vi "AeroTestBench.vi"() -> ()   [LabVIEW 2015]
uses:
  <vilib>/Utility/file.llb/Write To Spreadsheet File (DBL).vi
panel:
  in  "amp offset":dbl
  out "error out":errorcluster
  out "Attached":bool
  out "pulses in":i32
  out "ms":dbl
  out "Total Count:":i64
  out "Total Time (ms):":dbl
  out "Frequency (Hz):":dbl format="%#_6p"
  in  "Enabled":bool
  in  "Filter:":i32(ring)=1 items=["Zero Crossing"=1, "Logic Level"=2]
  in  "Timeout (ms):":i32=100
  in  "RPM:":i32 min=0 max=1 step=1
  in  "DataRate 2":i32(slide)=128 min=8 max=1000 step=8 scale=8.0..1000.0
  in  "stop":bool
  in  "Power":bool
  out "Amperage":dbl(knob) scale=0.0..80.0
  out "Voltage":dbl(knob) scale=0.0..30.0
  out "Enable":bool
  in  "Prop Blades":u8=2
  out "RPM":dbl(knob) scale=0.0..3000.0
  out "Power Electrical":dbl(knob) scale=0.0..1000.0
  out "Boolean 2":bool
  out "Effiency":dbl(knob) scale=0.0..100.0
  out "Power Mech":dbl(knob) scale=0.0..1000.0
  out "?":bool
  in  "Save data?":bool
  in  "Path":path
  in  "File Name":string
  out "Torque":dbl(knob) scale=-5.0..5.0
  out "Thrust":dbl(knob) scale=0.0..10.0
  in  "Gain":i32(ring)=6 items=["1"=1, "8"=2, "16"=3, "32"=4, "64"=5, "128"=6]
  in  "DataRate":i32(slide)=128 min=8 max=1000 step=8 scale=8.0..1000.0
  in  "Channel 3":i32(ring)=2 items=["0", "1", "2", "3"]
  in  "Channel 2":i32(ring)=1 items=["0", "1", "2", "3"]
  in  "Channel":i32(ring) items=["0", "1", "2", "3"]
  in  "Enable":bool
  out "Actives":i32
  out "Serial":i32
  out "Active":bool
  # "Arduino"
  # "(End with .csv)"
  # "(Should be 3+)"
  # "Phidgets"
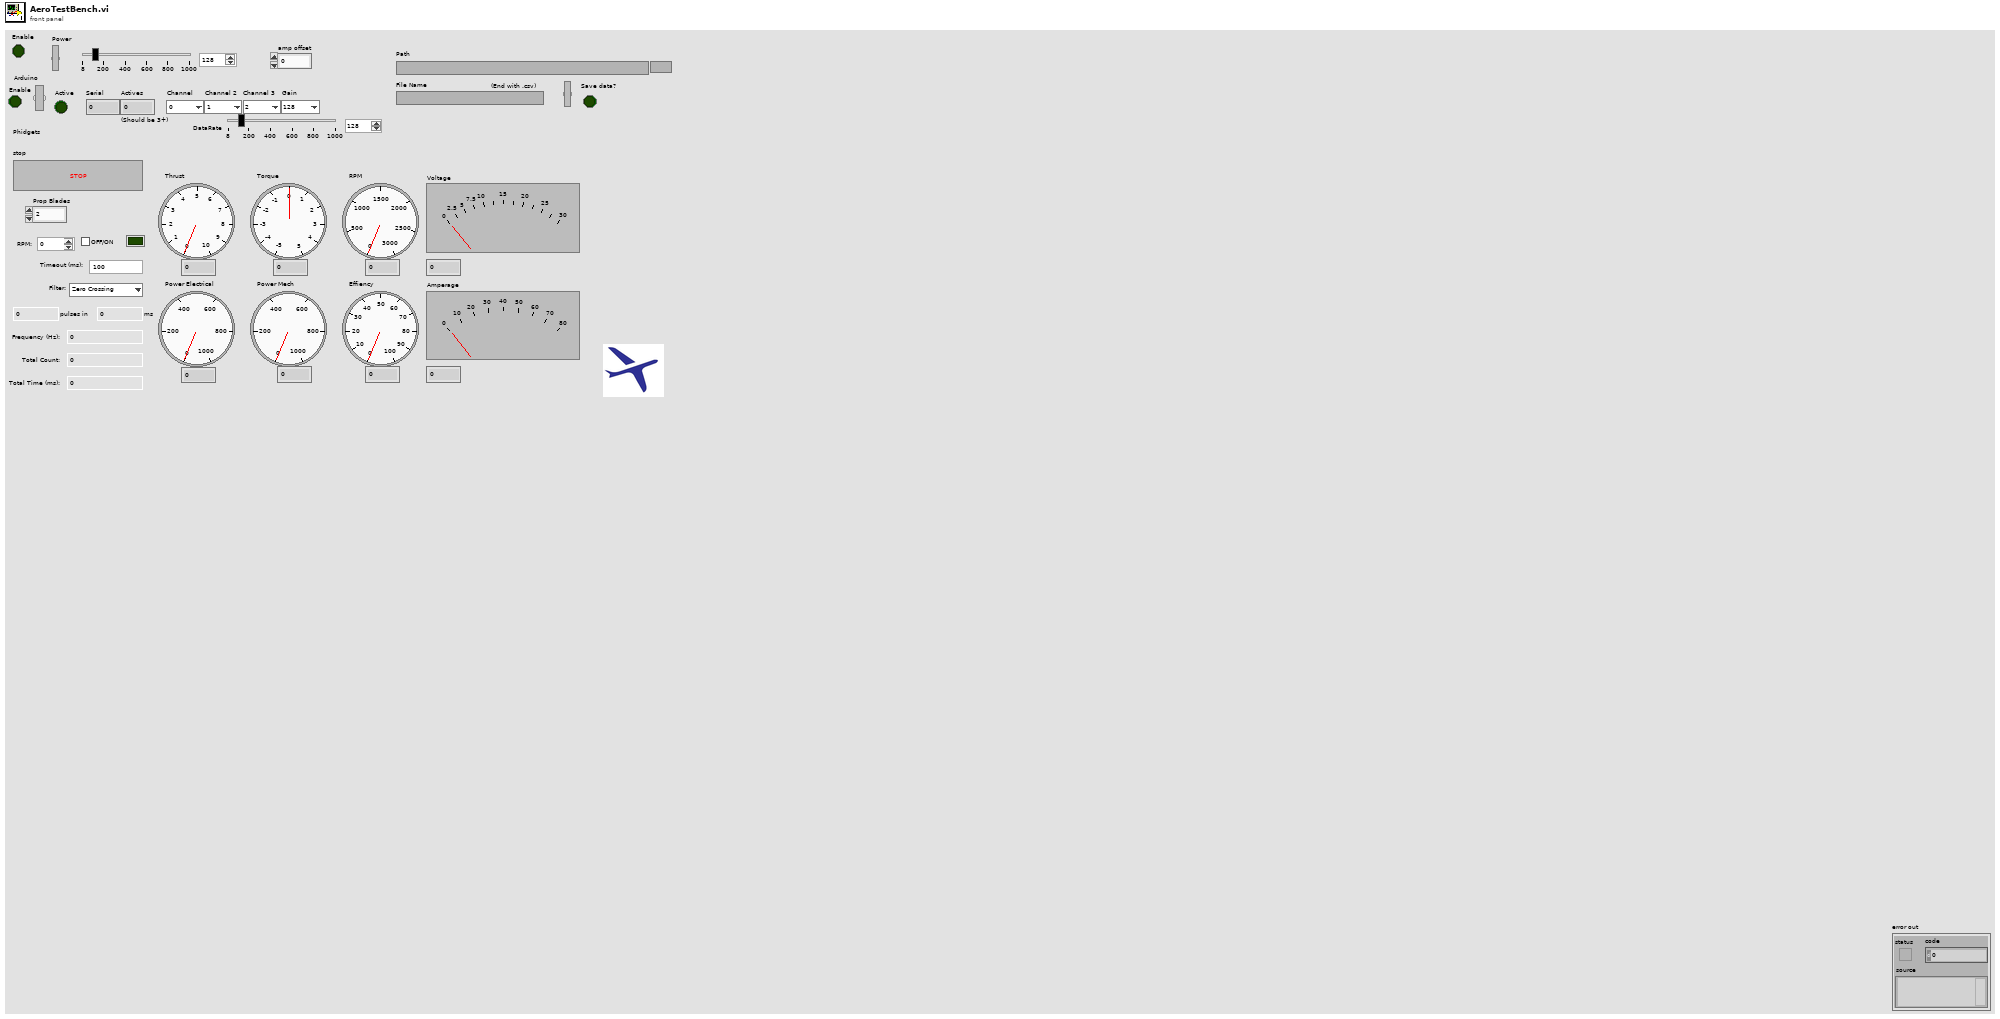
[diagram p1: front panel]
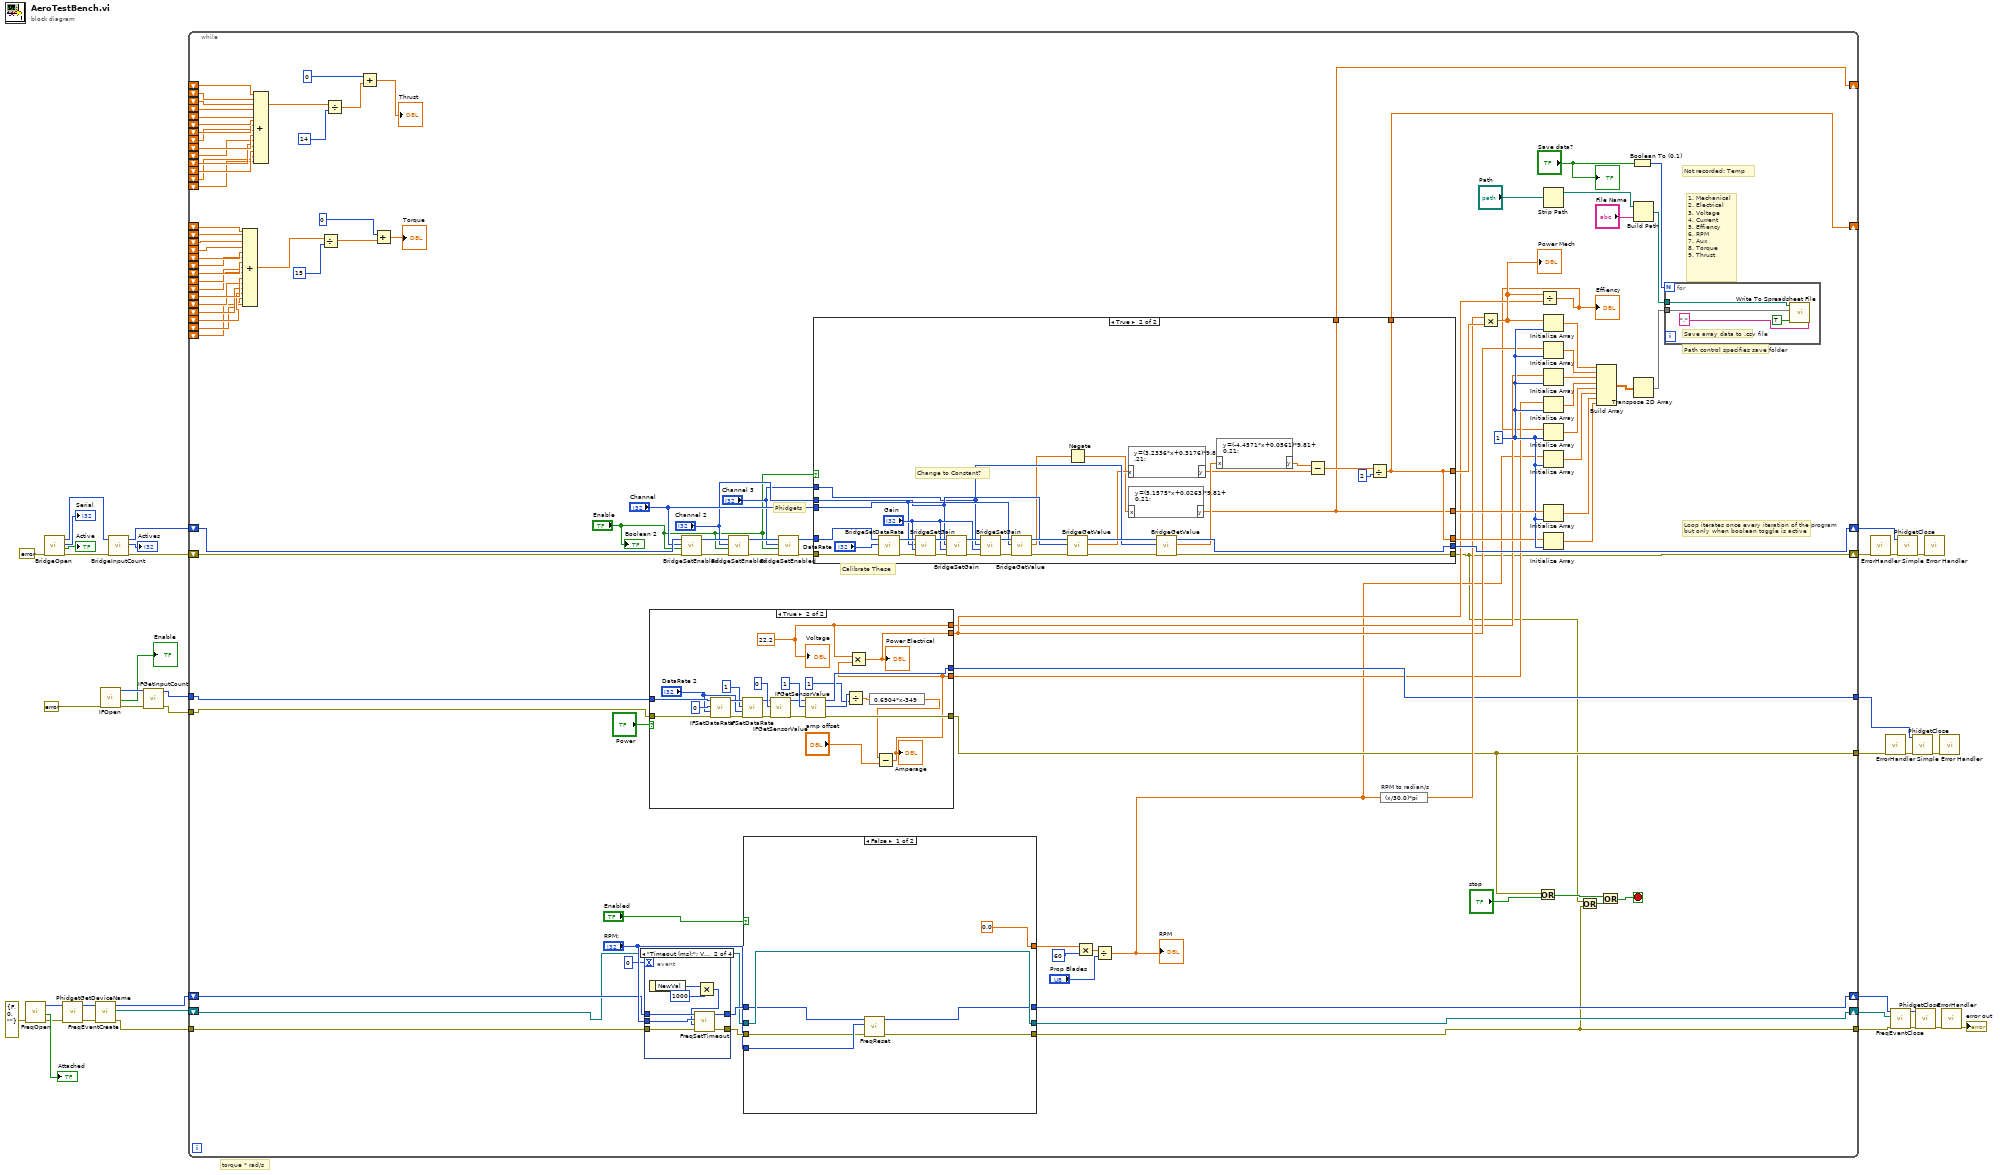
[diagram p0: block diagram]
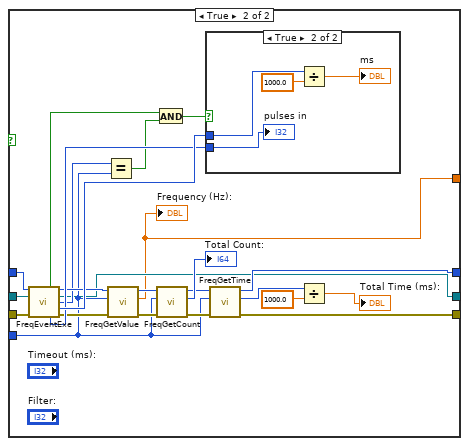
[diagram p2: hidden frame]
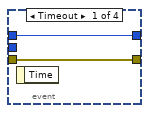
[diagram p4: hidden frame]
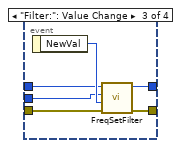
[diagram p5: hidden frame]
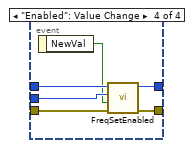
[diagram p6: hidden frame]
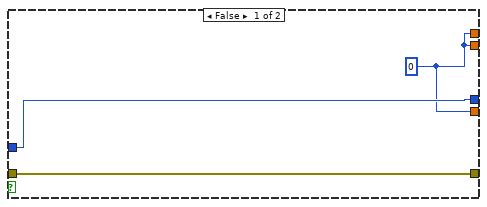
[diagram p7: hidden frame]
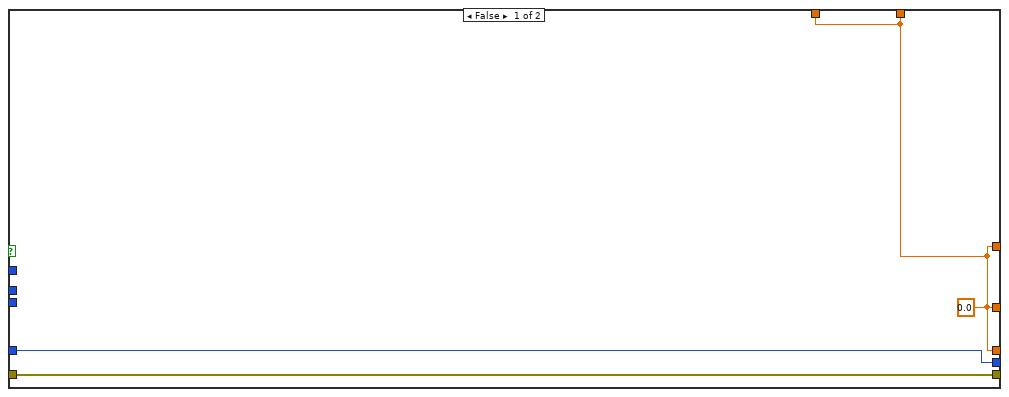
[diagram p8: hidden frame]
diagram:
  # "torque * rad/s"
  n1 = call "FreqOpen.vi"("error in (no error)"=errorcluster {"status"=FALSE, "code"=0, "source"=""}) -> ("error out"=w13:errorcluster, "Attached?"=→"Attached":bool, "Device Out"=w14:i64)  [unwired: 7 in, 1 out]
  n2 = call "BridgeOpen.vi"("error in (no error)"=errorcluster {"status"=FALSE, "code"=0, "source"=""} ("error constant")) -> ("error out"=w37:errorcluster, "Attached?"=→"Active":bool, "Serial Number Return"=→"Serial":i32, "Device Out"=w36:i64)  [unwired: 7 in]
  n3 = call "PhidgetGetDeviceName.vi"("error in"=w13, "Device In"=w14) -> ("error out"=w11:errorcluster, "Device Out"=w12:i64)  [unwired: 7 in, 1 out]
  n4 = call "FreqEventCreate.vi"("error in (no error)"=w11, "Device In"=w12) -> ("error out"=w10:errorcluster, "Event Registration Refnum Out"=w2:refnum<event-registration>, "Device Out"=w4:i64)  [unwired: 7 in]
  n5 = call "IFOpen.vi"("error in (no error)"=errorcluster {"status"=FALSE, "code"=0, "source"=""} ("error constant")) -> ("error out"=w26:errorcluster, "Attached?"=→"Enable":bool, "Device Out"=w25:i64)  [unwired: 7 in, 1 out]
  n6 = call "BridgeInputCount.vi"("error in (no error)"=w37, "Device In"=w36) -> ("error out"=w33:errorcluster, "Count"=→"Actives":i32, "Device Out"=w32:i64)  [unwired: 7 in]
  n7 = call "IFGetInputCount.vi"("error in (no error)"=w26, "Device In"=w25) -> ("error out"=w22:errorcluster, "Device Out"=w21:i64)  [unwired: 7 in, 1 out]
  n8 = while {
    shift-right: [w82] -> w28
    shift-left: w33 -> [w144]
    shift-right: [w133] -> w30
    shift-left: w32 -> [w143]
    tunnel: w22 -> [w105]
    tunnel: w21 -> [w104]
    tunnel: [w106] -> w18
    tunnel: [w107] -> w17
    tunnel: w10 -> [w94]
    tunnel: [w80] -> w5
    shift-right: [w92] -> w3
    shift-left: w4 -> [w93]
    shift-right: [w90] -> w1
    shift-left: w2 -> [w91]
    shift-right: [w74] -> _
    shift-left: _ -> [w79]
    shift-left: _ -> [w77]
    shift-left: _ -> [w78]
    shift-left: _ -> [w75]
    shift-left: _ -> [w76]
    shift-right: [w73] -> _
    shift-left: _ -> [w72]
    shift-left: _ -> [w71]
    shift-left: _ -> [w70]
    shift-left: _ -> [w69]
    shift-left: _ -> [w68]
    shift-left: _ -> [w57]
    shift-left: _ -> [w56]
    shift-left: _ -> [w55]
    shift-left: _ -> [w54]
    shift-left: _ -> [w53]
    shift-left: _ -> [w52]
    shift-left: _ -> [w51]
    shift-left: _ -> [w50]
    shift-left: _ -> [w49]
    shift-left: _ -> [w48]
    shift-left: _ -> [w47]
    shift-left: _ -> [w46]
    shift-left: _ -> [w45]
    shift-left: _ -> [w44]
    shift-left: _ -> [w43]
    shift-left: _ -> [w42]
    shift-left: _ -> [w41]
    shift-left: _ -> [w40]
    shift-left: _ -> [w39]
    stop <- w132 stop-if-true
    w113 = 1
    # "Not recorded: Temp"
    # "1. Mechanical\n2. Electrical\n3. Voltage\n4. Current\n5. Effiency \n6. RPM\n7. Aux\n8. Torque\n9. Thrust"
    # "Loop iterates once every iteration of the program\nbut only when boolean toggle is active"
    # "Path control specifies save folder"
    # "Calibrate These"
    # "Phidgets"
    n9 = Compound Arithmetic op=ADD(w72, w71, w70, w69, w68, w57, w56, w55, w54, w53, w52, w51, w50, w49, w48) -> (w65:dbl)
    n10 = Compound Arithmetic op=ADD(w79, w78, w77, w76, w75, w47, w46, w45, w44, w43, w42, w41, w40, w39) -> (w64:dbl)
    n11 = Divide(x=w65, y=15) -> (x/y=w62:dbl)
    n12 = Divide(x=w64, y=14) -> (x/y=w60:dbl)
    n13 = Add(x=0, y=w60) -> (x+y=→"Thrust":dbl)
    n14 = Add(x=0, y=w62) -> (x+y=→"Torque":dbl)
    n15 = event shown="[1] \"Timeout (ms):\": Value Change" {
      selector: _ -> [_ _ _ _]
      dyn-events: _ -> [_ _ _ _]
      timeout: 0 -> [_ _ _ _]
      tunnel: "RPM:" -> [_ w189 w192 w200]
      tunnel: w93 -> [w181 w188 w193 w201]
      tunnel: w94 -> [w180 w187 w194 w198]
      tunnel: [w180 w186 w190 w196] -> w97
      tunnel: [w181 w185 w191 w197] -> w98
      event Timeout {
        n16 = event-data() -> ()  [unwired: 1 in, 1 out]
      }
      event "Timeout (ms):": Value Change {
        n17 = event-data() -> ("NewVal"=w184:i32)  [unwired: 1 in]
        n18 = Multiply(x=w184, y=1000) -> (x*y=w182:i32)
        n19 = call "FreqSetTimeout.vi"("error in (no error)"=w187, "timeout"=w182, "index"=w189, "Device In"=w188) -> ("error out"=w186:errorcluster, "Device Out"=w185:i64)  [unwired: 5 in]
      }
      event "Filter:": Value Change {
        n20 = event-data() -> ("NewVal"=w195:i32)  [unwired: 1 in]
        n21 = call "FreqSetFilter.vi"("error in (no error)"=w194, "Filter"=w195, "index"=w192, "Device In"=w193) -> ("error out"=w190:errorcluster, "Device Out"=w191:i64)  [unwired: 5 in]
      }
      event "Enabled": Value Change {
        n22 = event-data() -> ("NewVal"=w199:bool)  [unwired: 1 in]
        n23 = call "FreqSetEnabled.vi"("error in (no error)"=w198, "SetEnabled"=w199, "index"=w200, "Device In"=w201) -> ("error out"=w196:errorcluster, "Device Out"=w197:i64)  [unwired: 5 in]
      }
    }
    n24 = case shown="True" "Power" {
      tunnel: [w204 w217] -> w106
      tunnel: [w203 w216] -> w107
      tunnel: w105 -> [w204 w219]
      tunnel: w104 -> [w203 w218]
      tunnel: [w202 w212] -> w103
      tunnel: [w202 w211] -> w102
      tunnel: [w202 w208] -> w101
      frame False {
        w202 = 0
      }
      frame True {
        w211 = 22.2
        n25 = call "IFSetDataRate.vi"("error in (no error)"=w219, "DataRate"="DataRate 2", "index"=0, "Device In"=w218) -> ("error out"=w223:errorcluster, "Device Out"=w222:i64)  [unwired: 5 in]
        n26 = call "IFSetDataRate.vi"("error in (no error)"=w223, "DataRate"="DataRate 2", "index"=1, "Device In"=w222) -> ("error out"=w221:errorcluster, "Device Out"=w220:i64)  [unwired: 5 in]
        n27 = call "IFGetSensorValue.vi"("error in (no error)"=w221, "index"=0, "Device In"=w220) -> ("error out"=w225:errorcluster, "Device Out"=w224:i64)  [unwired: 6 in, 1 out]
        n28 = call "IFGetSensorValue.vi"("error in (no error)"=w225, "index"=1, "Device In"=w224) -> ("error out"=w217:errorcluster, "Sensor Value"=w206:i32, "Device Out"=w216:i64)  [unwired: 6 in]
        n29 = Divide(x=w206, y=1) -> (x/y=w207:dbl)
        n30 = expression code="0.6904*x-349"(w207) -> (w210:dbl)
        n31 = Subtract(x=w210, y="amp offset") -> (x-y=w208:dbl)
        "Amperage" <- w208
        n32 = Multiply(x=w211, y=w208) -> (x*y=w212:dbl)
        "Power Electrical" <- w212
        "Voltage" <- w211
      }
    }
    n33 = call "BridgeSetEnabled.vi"("error in (no error)"=w144, "SetEnabled"="Enable", "index"="Channel", "Device In"=w143) -> ("error out"=w142:errorcluster, "Device Out"=w141:i64)  [unwired: 5 in]
    n34 = call "BridgeSetEnabled.vi"("error in (no error)"=w142, "SetEnabled"="Enable", "index"="Channel 2", "Device In"=w141) -> ("error out"=w140:errorcluster, "Device Out"=w139:i64)  [unwired: 5 in]
    n35 = case shown="False" "Enabled" {
      tunnel: w98 -> [w147 w175]
      tunnel: w91 -> [w151 w174]
      tunnel: w97 -> [w149 w173]
      tunnel: "RPM:" -> [w150 w159]
      tunnel: [w146 w155] -> w92
      tunnel: [w151 w154] -> w90
      tunnel: [w148 w153] -> w80
      tunnel: [0.0 w152] -> w87
      frame False {
        n36 = call "FreqReset.vi"("error in (no error)"=w149, "index"=w150, "Device In"=w147) -> ("error out"=w148:errorcluster, "Device Out"=w146:i64)  [unwired: 6 in]
      }
      frame True {
        n37 = call "FreqEventExe.vi"("Device In"=w175, "Event Registration Refnum In"=w174, "error in (no error)"=w173) -> ("Event?"=w169:bool, "Device Out"=w167:i64, "Event Registration Refnum Out"=w154:refnum<event-registration>, "index"=w164:i32, "time"=w171:i32, "counts"=w170:i32, "error out"=w166:errorcluster)  [unwired: 6 in]
        n38 = Equal?(x=w164, y=w159) -> (x = y?=w168:bool)
        n39 = call "FreqGetValue.vi"("error in (no error)"=w166, "index"=w159, "Device In"=w167) -> ("error out"=w163:errorcluster, "Frequency"=w152:dbl, "Device Out"=w165:i64)  [unwired: 5 in]
        "Frequency (Hz):" <- w152
        n40 = And(x=w169, y=w168) -> (x .and. y?=w172:bool)
        n41 = call "FreqGetCount.vi"("error in (no error)"=w163, "index"=w159, "Device In"=w165) -> ("error out"=w161:errorcluster, "Count"=→"Total Count:":i64, "Device Out"=w160:i64)  [unwired: 5 in]
        n42 = case shown="True" w172 {
          tunnel: w171 -> [_ w177]
          tunnel: w170 -> [_ w179]
          frame False {
          }
          frame True {
            n43 = Divide(x=w177, y=1000.0) -> (x/y=→"ms":dbl)
            "pulses in" <- w179
          }
        }
        n44 = call "FreqGetTime.vi"("error in (no error)"=w161, "index"=w159, "Device In"=w160) -> ("error out"=w153:errorcluster, "Time"=w158:i64, "Device Out"=w155:i64)  [unwired: 5 in]
        n45 = Divide(x=w158, y=1000.0) -> (x/y=→"Total Time (ms):":dbl)
      }
    }
    n46 = call "BridgeSetEnabled.vi"("error in (no error)"=w140, "SetEnabled"="Enable", "index"="Channel 3", "Device In"=w139) -> ("error out"=w137:errorcluster, "Device Out"=w138:i64)  [unwired: 5 in]
    n47 = case shown="True" "Enable" {
      tunnel: w138 -> [w233 w265]
      tunnel: w137 -> [w234 w264]
      tunnel: "Channel" -> [_ w253]
      tunnel: "Channel 2" -> [_ w250]
      tunnel: "Channel 3" -> [_ w247]
      tunnel: [w233 w246] -> w133
      tunnel: [w234 w245] -> w82
      tunnel: [w232 w235] -> w130
      tunnel: [w232 w236] -> w112
      tunnel: [w232 w235] -> w117
      tunnel: [w232 w236] -> w74
      tunnel: [w232 w235] -> w73
      frame False {
        w232 = 0.0
      }
      frame True {
        # "Change to Constant?"
        n48 = call "BridgeSetDataRate.vi"("error in (no error)"=w264, "DataRate"="DataRate", "Device In"=w265) -> ("error out"=w262:errorcluster, "Device Out"=w261:i64)  [unwired: 6 in]
        n49 = call "BridgeSetGain.vi"("error in (no error)"=w262, "gain"="Gain", "index"=w253, "Device In"=w261) -> ("error out"=w260:errorcluster, "Device Out"=w259:i64)  [unwired: 5 in]
        n50 = call "BridgeSetGain.vi"("error in (no error)"=w260, "gain"="Gain", "index"=w250, "Device In"=w259) -> ("error out"=w258:errorcluster, "Device Out"=w257:i64)  [unwired: 5 in]
        n51 = call "BridgeSetGain.vi"("error in (no error)"=w258, "gain"="Gain", "index"=w247, "Device In"=w257) -> ("error out"=w255:errorcluster, "Device Out"=w254:i64)  [unwired: 5 in]
        n52 = call "BridgeGetValue.vi"("error in (no error)"=w255, "index"=w253, "Device In"=w254) -> ("error out"=w251:errorcluster, "value"=w237:dbl, "Device Out"=w252:i64)  [unwired: 5 in]
        n53 = Negate(x=w237) -> (-x=w238:dbl)
        n54 = call "BridgeGetValue.vi"("error in (no error)"=w251, "index"=w250, "Device In"=w252) -> ("error out"=w249:errorcluster, "value"=w244:dbl, "Device Out"=w248:i64)  [unwired: 5 in]
        n55 = formula code="y=(3.2336*x+0.3176)*9.81+0.21;"("x"=w244) -> ("y"=w240:dbl)
        n56 = formula code="y=(5.1575*x+0.0263)*9.81+0.21;"("x"=w238) -> ("y"=w236:dbl)
        n57 = call "BridgeGetValue.vi"("error in (no error)"=w249, "index"=w247, "Device In"=w248) -> ("error out"=w245:errorcluster, "value"=w243:dbl, "Device Out"=w246:i64)  [unwired: 5 in]
        n58 = formula code="y=(-4.4571*x+0.0561)*9.81+0.21;"("x"=w243) -> ("y"=w239:dbl)
        n59 = Subtract(x=w239, y=w240) -> (x-y=w242:dbl)
        n60 = Divide(x=w242, y=2) -> (x/y=w235:dbl)
      }
    }
    n61 = Multiply(x=w87, y=60) -> (x*y=w89:dbl)
    n62 = Divide(x=w89, y="Prop Blades") -> (x/y=w85:dbl)
    "RPM" <- w85
    n63 = expression code="(x/30.0)*pi" "RPM to radian/s"(w85) -> (w110:dbl)
    n64 = Multiply(x=w110, y=w117) -> (x*y=w115:dbl)
    "Power Mech" <- w115
    n65 = Or(x=w106, y="stop") -> (x .or. y?=w131:bool)
    n66 = Divide(x=w115, y=w103) -> (x/y=w100:dbl)
    "Effiency" <- w100
    n67 = Strip Path(path="Path") -> (stripped path=w128:path)  [unwired: 1 out]
    n68 = Initialize Array(w115, w113) -> (w114:dbl[])
    n69 = Initialize Array(w103, w113) -> (w116:dbl[])
    n70 = Initialize Array(w102, w113) -> (w119:dbl[])
    n71 = Initialize Array(w101, w113) -> (w121:dbl[])
    n72 = Initialize Array(w100, w113) -> (w122:dbl[])
    n73 = Initialize Array(w85, w113) -> (w123:dbl[])
    n74 = Initialize Array(w130, w113) -> (w84:dbl[])
    n75 = Initialize Array(w112, w113) -> (w83:dbl[])
    n76 = Or(x=w82, y=w80) -> (x .or. y?=w81:bool)
    n77 = Build Array(w114, w116, w119, w121, w122, w123, w84, w83) -> (w124:dbl[][])
    n78 = Or(x=w131, y=w81) -> (x .or. y?=w132:bool)
    n79 = Boolean To (0,1)(Boolean="Save data?") -> (0, 1=w126:i16)
    n80 = Build Path(base path=w128, name or relative path="File Name") -> (appended path=w120:path)
    n81 = Transpose 2D Array(2D array=w124) -> (transposed array=w118:dbl[][])
    n82 = for {
      N: w126 -> [_]
      tunnel: w120 -> [w229]
      tunnel: w118 -> [w228]
      # "Save array data to .csv file"
      n83 = call-poly <vilib>:"Write To Spreadsheet File.vi"("delimiter (\\t)"=",", "append to file? (new file:F)"=TRUE, "2D data"=w228, "file path (dialog if empty)"=w229) -> ()  [unwired: 4 in, 1 out]
    }
    "?" <- "Save data?"
    "Boolean 2" <- "Enable"
  }
  n84 = call "ErrorHandler.vi"("error in"=w28) -> ("error out"=w29:errorcluster)  [unwired: 9 in, 1 out]
  n85 = call "ErrorHandler.vi"("error in"=w18) -> ("error out"=w20:errorcluster)  [unwired: 9 in, 1 out]
  n86 = call "FreqEventClose.vi"("error in (no error)"=w5, "Event Registration Refnum In"=w1, "Device In"=w3) -> ("error out"=w6:errorcluster, "Device Out"=w7:i64)  [unwired: 7 in]
  n87 = call "PhidgetClose.vi"("error in"=w29, "Device In"=w30) -> ("error out"=w27:errorcluster)  [unwired: 9 in]
  n88 = call "PhidgetClose.vi"("error in"=w20, "Device In"=w17) -> ("error out"=w19:errorcluster)  [unwired: 9 in]
  n89 = call "PhidgetClose.vi"("error in"=w6, "Device In"=w7) -> ("error out"=w9:errorcluster)  [unwired: 9 in]
  n90 = call <vilib>:"Simple Error Handler.vi"("error in (no error)"=w27) -> ()  [unwired: 4 in, 5 out]
  n91 = call <vilib>:"Simple Error Handler.vi"("error in (no error)"=w19) -> ()  [unwired: 4 in, 5 out]
  n92 = call "ErrorHandler.vi"("error in"=w9) -> ("error out"=→"error out":errorcluster)  [unwired: 9 in, 1 out]
